vi "Recursive List.vi"() -> ()   [LabVIEW 2011]
panel:
  out "Folders":path[](array[path])
  out "Files":path[](array[path])
  out "Error Out":errorcluster
  in  "Error in":errorcluster
  in  "Start Path\n(empty - Prompt)":path
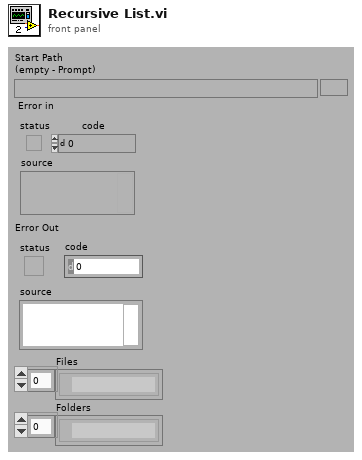
[diagram p1: front panel]
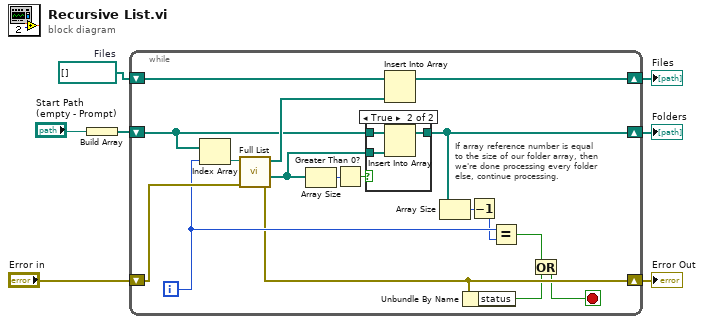
[diagram p0: block diagram]
diagram:
  w4 = path[] []  # Files
  n1 = Build Array("Start Path\n(empty - Prompt)") -> (w6:path[])
  n2 = while {
    shift-right: [w16] -> w1
    shift-left: w6 -> [w19]
    shift-right: [w14] -> w3
    shift-left: "Error in" -> [w23]
    shift-right: [w20] -> w2
    shift-left: w4 -> [w22]
    i -> [w18]
    stop <- w11 stop-if-true
    # "If array reference number is equal\nto the size of our folder array, then\nwe're done processing every folder\nelse, continue processing."
    n3 = Index Array(array=w19, index=w18) -> (element=w24:path)
    n4 = call "Full List.vi"("Error in"=w23, "Start Path\n(empty - Prompt)"=w24) -> ("Error out"=w14:errorcluster, "Folders"=w8:path[], "Files"=w21:path[])  [unwired: 3 out]
    n5 = Array Size(array=w8) -> (size(s)=w9:i32)
    n6 = Greater Than 0?(x=w9) -> (x > 0?=w10:bool)
    n7 = case shown="True" w10 {
      tunnel: w8 -> [_ w28]
      tunnel: w19 -> [w25 w27]
      tunnel: [w25 w26] -> w16
      frame False {
      }
      frame True {
        n8 = Insert Into Array(array=w27, new element=w28) -> (w26:path[])  [unwired: 1 in]
      }
    }
    n9 = Insert Into Array(array=w22, new element=w21) -> (w20:path[])  [unwired: 1 in]
    n10 = Array Size(array=w16) -> (size(s)=w17:i32)
    n11 = Unbundle By Name(w14) -> ("status"=w13:bool)
    n12 = Decrement(x=w17) -> (x-1=w15:i32)
    n13 = Equal?(x=w18, y=w15) -> (x = y?=w12:bool)
    n14 = Or(x=w12, y=w13) -> (x .or. y?=w11:bool)
  }
  "Error Out" <- w3
  "Files" <- w2
  "Folders" <- w1
